vi "Simulation.vi"() -> ()   [LabVIEW 2014]
uses:
  <vilib>/Simulation/Implementation/XNodeFramework/SimXNode/SimX.xnode
  <vilib>/Simulation/Implementation/Shared/SIMSCR Execution Mode.ctl
  <vilib>/Simulation/Scripting/Companion Diagram/SimConfigNode/_simSolvers.ctl
  <vilib>/Simulation/Scripting/Companion Diagram/SimConfigNode/SimParams.ctl
  <vilib>/Simulation/Scripting/Companion Diagram/SimConfigNode/SimDog.xnode
  <vilib>/Simulation/SignalArithmetic/Implementation/NILVSim Gain.llb/SIM Gain (scalar).vi
  <vilib>/Simulation/SignalArithmetic/Implementation/NILVSim Gain.llb/SIM Gain (vector).vi
  <vilib>/Simulation/Utility/Implementation/SIM Halt.vi
  Nichtlineares Pendelmodell Sub.vi
  LabView/Beobachter/Nichtlinearer Beobachter.vi
  <vilib>/addons/Control Design/_Model Construction/Model Typedefs.llb/CD General Elements.ctl
  <vilib>/addons/Control Design/_Model Construction/NI_LinSys_Model Typedefs.lvlib
  <vilib>/addons/Control Design/_Model Construction/Model Typedefs.llb/CD State Space Model (MIMO).ctl
  <vilib>/addons/Control Design/_State Feedback Control/State Feedback Control.llb/CD Linear Quadratic Regulator.vi
  <vilib>/addons/Control Design/_State Feedback Control/NI_CD_State Feedback Control.lvlib
  <vilib>/addons/Control Design/_State Feedback Control/State Feedback Control.llb/State Feedback Control SubVis/cd_Linear Quadratic Regulator.vi
  <vilib>/addons/Control Design/_Utility/NI_CD_Model Viewer.lvlib
  <vilib>/addons/Control Design/_Utility/Model Viewer.llb/Model Viewer SubVI/cd_Draw State-Space Equation (SS).vi
  <vilib>/addons/Control Design/_Model Construction/NI_LinSys_Model Creation.lvlib
  <vilib>/addons/Control Design/_Model Construction/Model Creation.llb/Model Creation SubVI/cd_Create State Space Model.vi
  <vilib>/Simulation/SignalArithmetic/Implementation/NILVSim Gain.llb/SIM Gain (vector,MatrixGain).vi
  <vilib>/Simulation/ContinuousLinear/Implementation/NILVSim State Space.llb/SIM State Space (CD).vi
  <vilib>/Simulation/Nonlinear/Implementation/NILVSim Saturation.llb/SIM Saturation (scalar).vi
panel:
  out "State-Space Equation":picture
  in  "Winkelg._t0":dbl
  in  "WG Regler":enum16{"geschätzt", "simuliert"}(ring)
  in  "WG Aufschw.":enum16{"geschätzt", "simuliert"}(ring)=enum."simuliert"
  out "geschätzt+gefiltert":dbl
  out "Cruise mode":dbl(graph)
  out "Regler":i16(graph)
  in  "< Winkelgeschwindigkeit (rad)":dbl=1.0
  in  ">Winkel (Grad) AUS":dbl=15.0
  in  "<Winkel (Grad) EIN":dbl=10.0
  in  "k_cein (EIN)":dbl=1.05
  in  "k_caus(AUS)":dbl=0.75
  in  "k_eo (Energieoffset)":dbl=1.05
  in  "k_ce (Energiezufuhr)":dbl=2.5
  out "E kin":dbl(graph)
  out "E pot":dbl(graph)
  out "E gesamt":dbl(graph)
  in  "Position_t0 (m)":dbl
  out "Kraft in N":dbl=33.7
  out "winkelgesch Geschätzt":dbl=9.681355067256998
  out "Winkelgesch. Simuliert":dbl=9.66876102656205
  out "Winkel  (rad)":dbl=2.875919721526653
  out "Geschwindigkeit":dbl=-0.30635447737283783
  out "Position":dbl=-291.9143512126312
  out "Regler EIN":bool
  in  "k_v (velocity well)":dbl=1.0
  in  "k_x (cart well)":dbl=2.5
  in  "k_e (Energiezufuhr)":dbl=2.5
  in  "Aufschwingen":bool=TRUE
  in  "Strecke":T1(ring)
  out "Position (mm)":cluster{"output":dbl, "output":dbl}(graph)={"output"=0.0, "output"=-291.9143512126312}
  out "Winkel (Grad)":cluster{"Winkelgesch":dbl}(graph)={"Winkelgesch"=164.77806226191623}
  out "Kraft (N)":dbl(graph)=33.7
  out "Geschwindigkeit":dbl(graph)=-0.30635447737283783
  out "Winkelgeschwindigkeit":cluster{"Winkelgesch":dbl, "x4_":dbl}(graph)={"Winkelgesch"=9.66876102656205, "x4_"=9.681355067256998}
  out "K":dbl[][](array[numeric])=[[-99.99999999999996, -103.97875304957287, -705.5157122075409, -139.58745173214928]] format="%.2f"
  in  "Q":dbl[][](array[numeric])=[[100.0, 0.0, 0.0, 0.0], [0.0, 1.0, 0.0, 0.0], [0.0, 0.0, 100.0, 0.0], [0.0, 0.0, 0.0, 1.0]] format="%.2f"
  in  "R":dbl[][](array[numeric])=[[0.01]] format="%.2f"
  in  "Regler":bool=TRUE
  in  "Winkel_t0 (Grad)":dbl=180.0
  in  "Sollwert Amplitude (mm)":dbl
  in  "Stop Button":bool
  # "Anfangswerte"
  # "Aufschwingparameter"
  # "Umschalten auf Cruise Mode. Energiegrenzen"
  # "Umschalten auf Regler"
  # "LQR Regler"
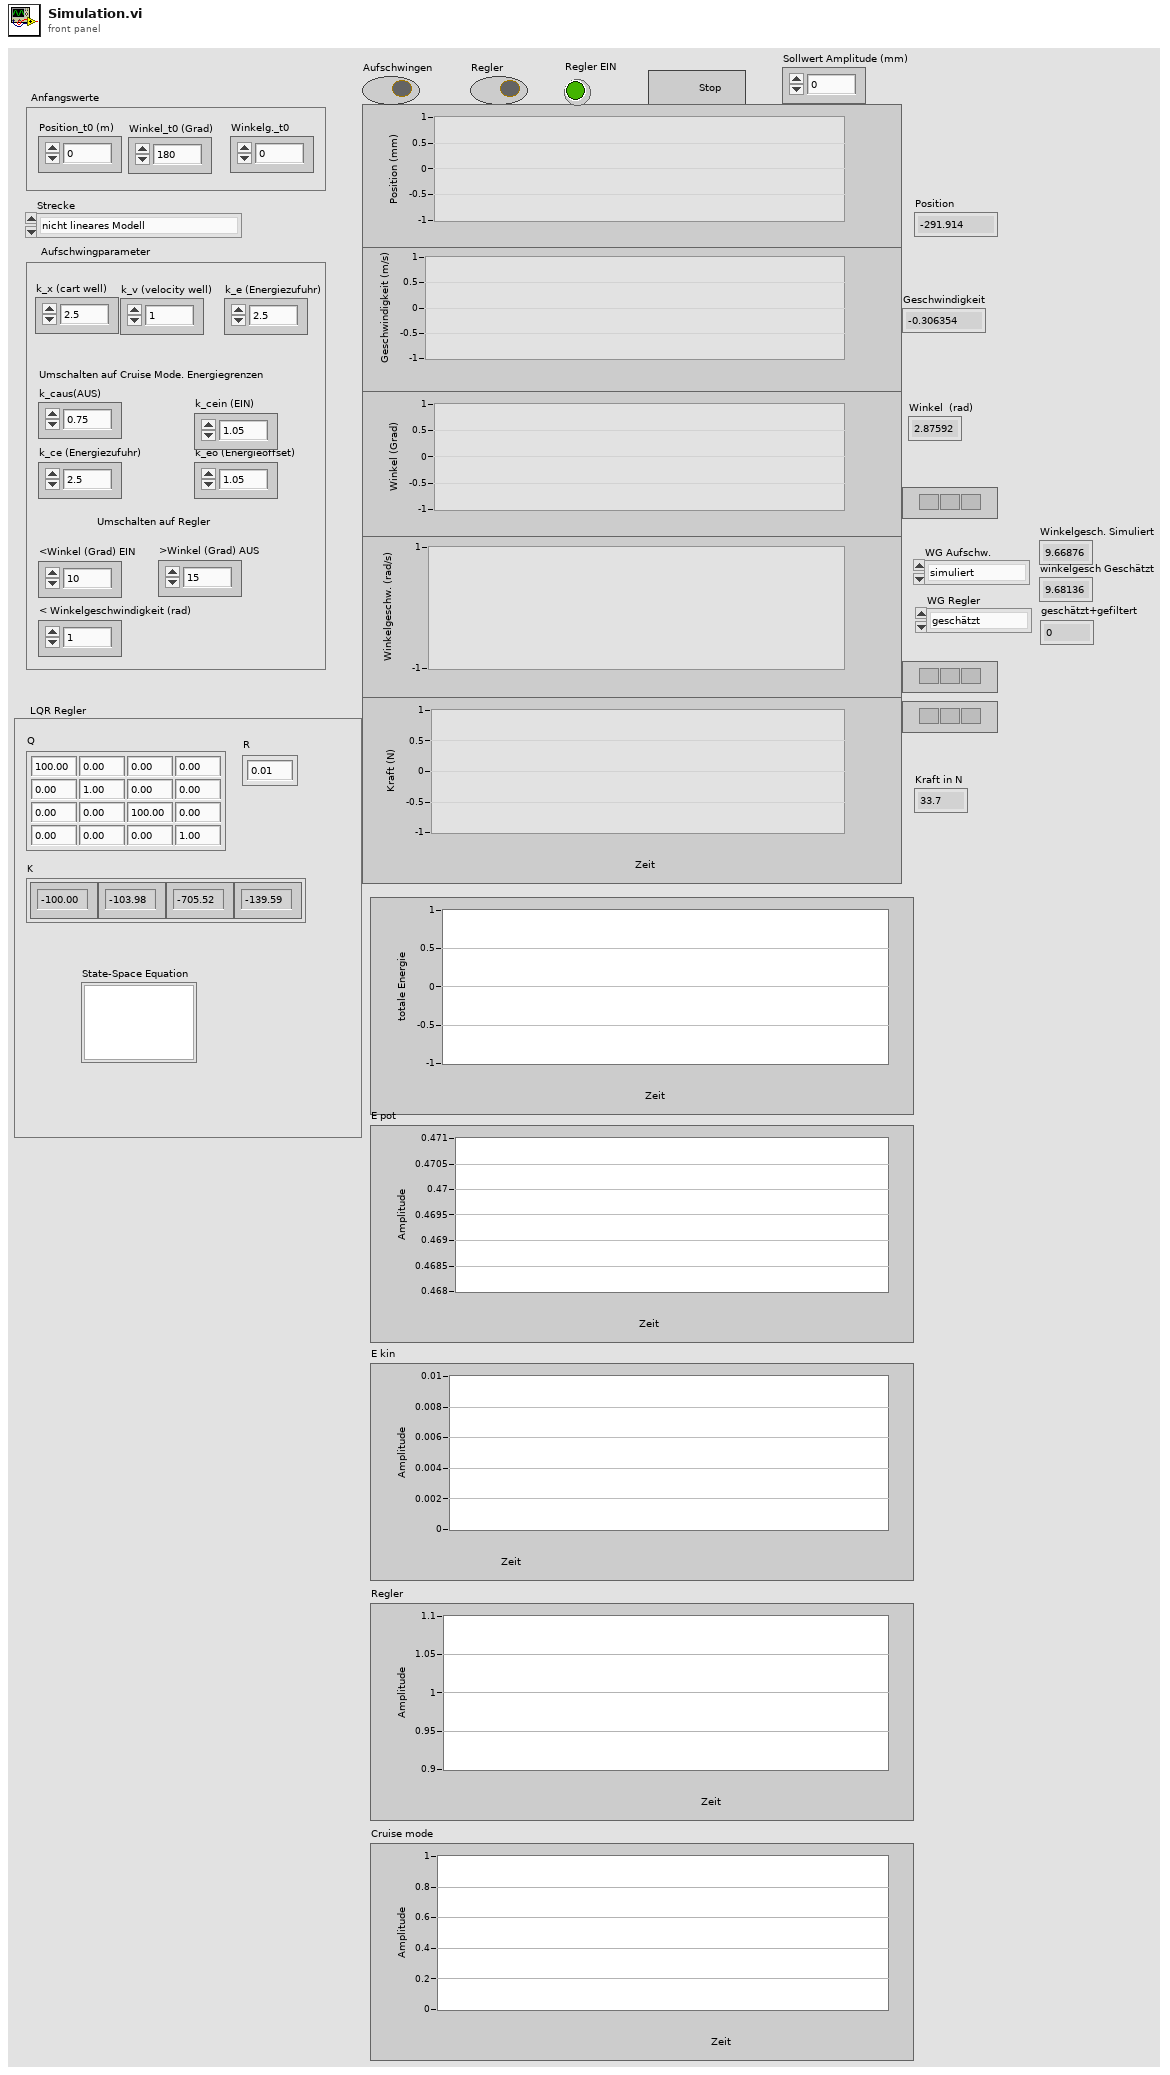
[diagram p1: front panel]
types:
  T1 = enum16{"nicht lineares Modell", "lineares Modell"}
  T2 = typedef "NI_LinSys_Model Typedefs.lvlib/CD State Space Model (MIMO).ctl" = cluster{"properties":T3, "A":dbl[][], "B":dbl[][], "C":dbl[][], "D":dbl[][], "StateNames":string[], "Transport Delay":dbl[][]}
  T3 = typedef "NI_LinSys_Model Typedefs.lvlib/CD General Elements.ctl" = cluster{"Model name":string, "Input names":string[], "Output names":string[], "Input Delays":dbl[], "Output Delays":dbl[], "Sampling Time":dbl, "Notes":string}
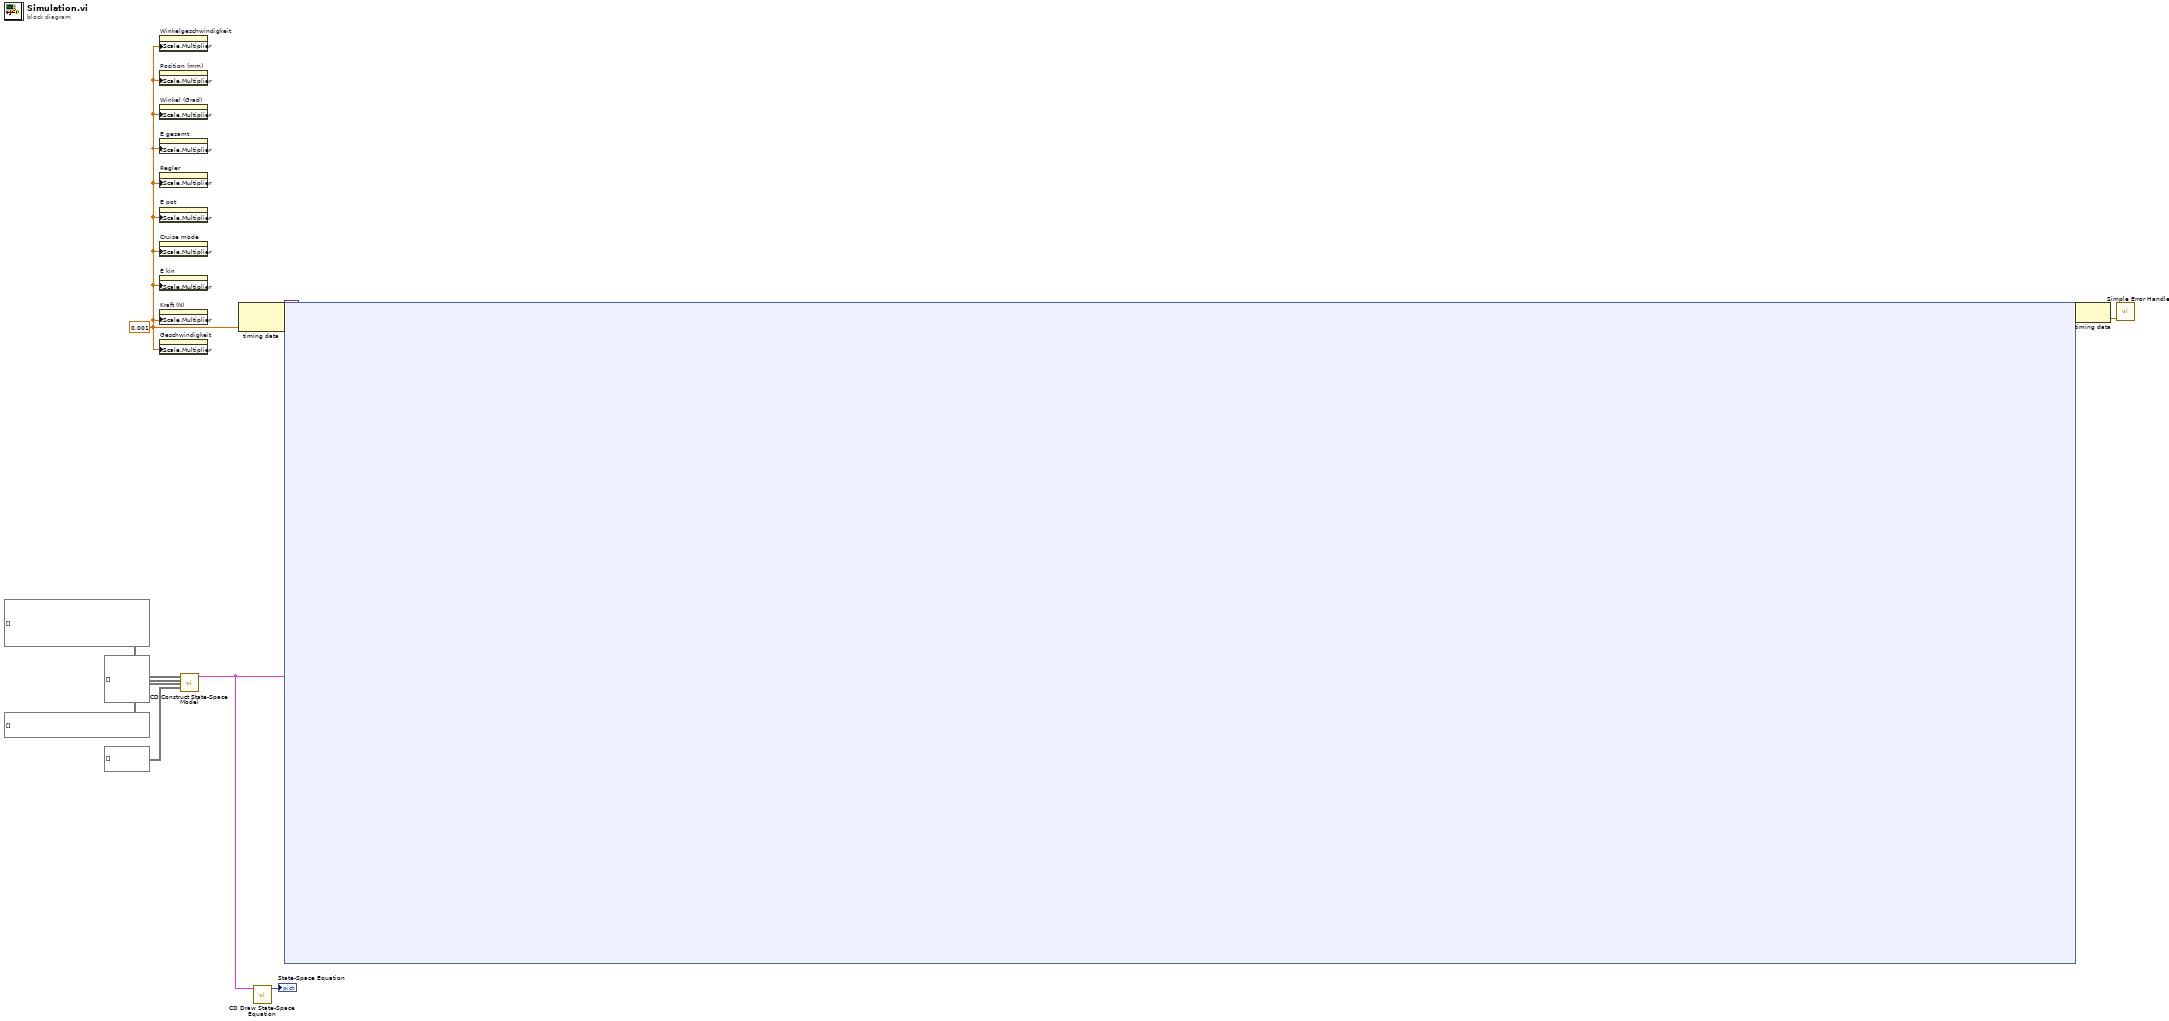
[diagram p0: block diagram]
diagram:
  w2 = 0.001 ("Step Size (s)")
  n1 = property on="Winkelgeschwindigkeit" class="SVDiagr (strikt)"("XScale.Multiplier"=w2) -> ()  [unwired: 2 in, 2 out]
  n2 = property on="Position (mm)" class="SVDiagr (strikt)"("XScale.Multiplier"=w2) -> ()  [unwired: 2 in, 2 out]
  n3 = property on="Winkel (Grad)" class="SVDiagr (strikt)"("XScale.Multiplier"=w2) -> ()  [unwired: 2 in, 2 out]
  n4 = property on="E gesamt" class="SVDiagr (strikt)"("XScale.Multiplier"=w2) -> ()  [unwired: 2 in, 2 out]
  n5 = property on="Regler" class="SVDiagr (strikt)"("XScale.Multiplier"=w2) -> ()  [unwired: 2 in, 2 out]
  n6 = property on="E pot" class="SVDiagr (strikt)"("XScale.Multiplier"=w2) -> ()  [unwired: 2 in, 2 out]
  n7 = property on="Cruise mode" class="SVDiagr (strikt)"("XScale.Multiplier"=w2) -> ()  [unwired: 2 in, 2 out]
  n8 = property on="E kin" class="SVDiagr (strikt)"("XScale.Multiplier"=w2) -> ()  [unwired: 2 in, 2 out]
  n9 = property on="Kraft (N)" class="SVDiagr (strikt)"("XScale.Multiplier"=w2) -> ()  [unwired: 2 in, 2 out]
  n10 = property on="Geschwindigkeit" class="SVDiagr (strikt)"("XScale.Multiplier"=w2) -> ()  [unwired: 2 in, 2 out]
  n11 = call-poly <vilib>:"CD Construct State-Space Model.vi"("A"=void[][] [], "B"=void[][] [], "C"=void[][] [], "D"=void[][] []) -> ("State-Space Model"=w3:T2)  [unwired: 10 in, 1 out]
  n12 = node-c288(w2) -> (w10:variant)  [unwired: 1 in]
  n13 = call-poly <vilib>:"CD Draw State-Space Equation.vi"("State-Space Model"=w3) -> ("Equation"=→"State-Space Equation":picture)  [unwired: 8 in, 2 out]
  n14 = node-c254 ("Control & Simulation Loop")(w10, w3) -> (w9:variant)
  n15 = node-c288(w9) -> (w8:errorcluster)
  n16 = call <vilib>:"Simple Error Handler.vi"("error in (no error)"=w8) -> ()  [unwired: 4 in, 5 out]
